vi "BezierGeneratorRev2Trans.vi"(1 "RobotY":dbl, 2 "RobotX":dbl, 3 "DeltaYaw":dbl, 4 "RobotOrientation":dbl=70.0, 5 "DeltaY":dbl=60.0, 6 "DeltaX":dbl=60.0) -> (0 "RobotNeededPathData":T1={"Path"=[], "MaxVel"=80.0, "MaxAccel"=100.0, "Backwards?"=FALSE, "PointSpacing"=6.0, "LookaheadDist"=13.0, "Speed/Curve"=1.8, "SlowDistanceAtEnd"=0.0, "SlowSpeed"=0.0, "MaxDeAccel"=80.0} {"SlowSpeed" format="%#_13g"; "SlowDistanceAtEnd" format="%#_13g"; "Speed/Curve" format="%#_13g"})   [LabVIEW 2018]
uses:
  FRC-2019-master/FRC-2019-master/Dawgma Programming Library/Controls/PurePursuit/RobotNeededPathData.ctl
panel:
  in  "SlowSpeed":dbl
  in  "SlowDistanceAtEnd":dbl
  in  "Speed/Curve":dbl=1.8
  in  "LookaheadDist":dbl=13.0
  in  "PointSpacing":dbl=6.0
  in  "MaxDeaccel":dbl=80.0
  in  "MaxAccel":dbl=100.0
  in  "MaxVel":dbl=80.0
  out "Curve":cluster{"X":dbl, "Y":dbl}[](graph)
  out "waypoints":cluster{dbl[], dbl[]}(graph)
  in  "TrajPointoffset":dbl=12.0
  in  "TargetOffset":dbl=12.0
  in  "Path":cluster{"x":dbl, "y":dbl}[](array[cluster])=[{"x"=0.0, "y"=0.0}, {"x"=0.0, "y"=0.0}, {"x"=0.0, "y"=0.0}, {"x"=0.0, "y"=0.0}]
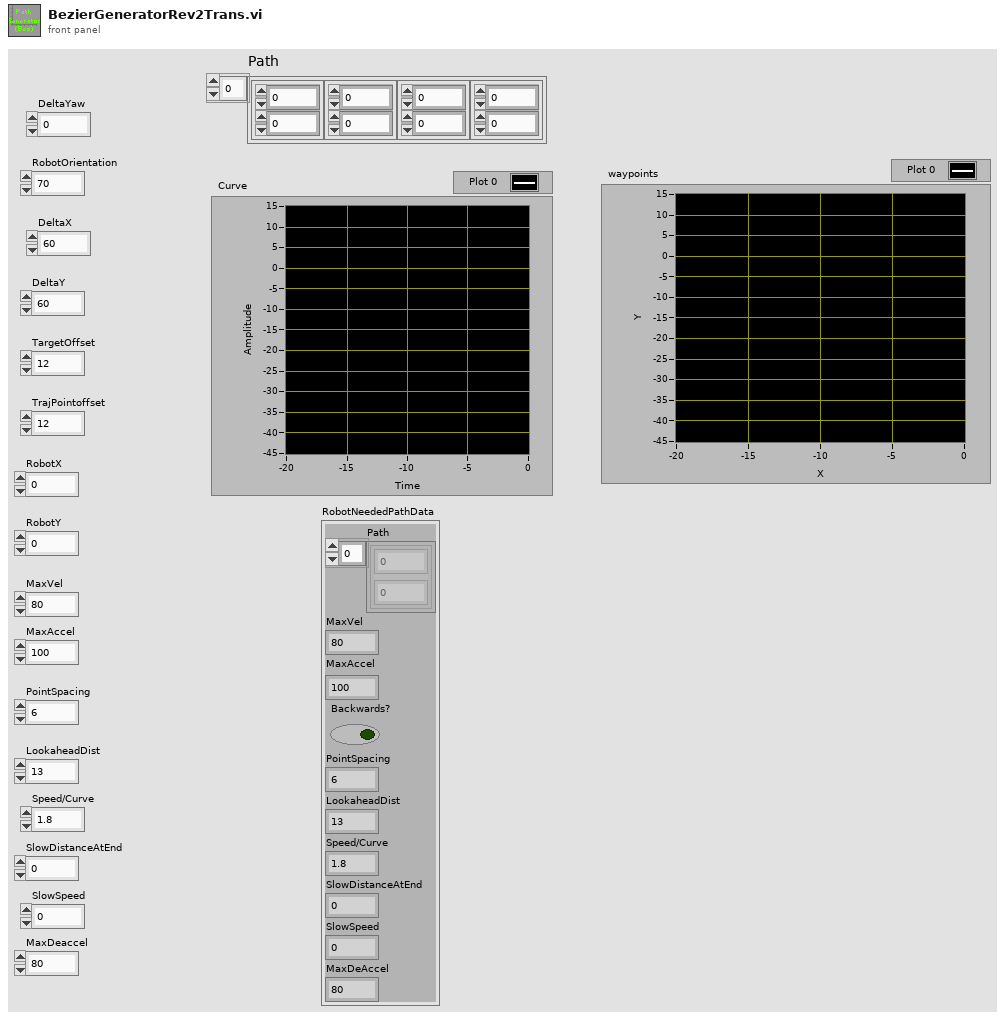
[diagram p1: front panel]
types:
  T1 = typedef "RobotNeededPathData.ctl" = cluster{"Path":cluster{dbl, dbl}[], "MaxVel":dbl, "MaxAccel":dbl, "Backwards?":bool, "PointSpacing":dbl, "LookaheadDist":dbl, "Speed/Curve":dbl, "SlowDistanceAtEnd":dbl, "SlowSpeed":dbl, "MaxDeAccel":dbl}
  T2 = cluster{"DeltaX":dbl, "DeltaY":dbl, "RobotOrientation":dbl, "TrajPointoffset":dbl, "TargetOffset":dbl, "DeltaYaw":dbl, "RobotX":dbl, "RobotY":dbl}
  T3 = cluster{cluster{"xP":dbl, "yP":dbl}[], "MaxVel":dbl, "MaxAccel":dbl, bool, "PointSpacing":dbl, "LookaheadDist":dbl, "Speed/Curve":dbl, "SlowDistanceAtEnd":dbl, "SlowSpeed":dbl, "MaxDeaccel":dbl}
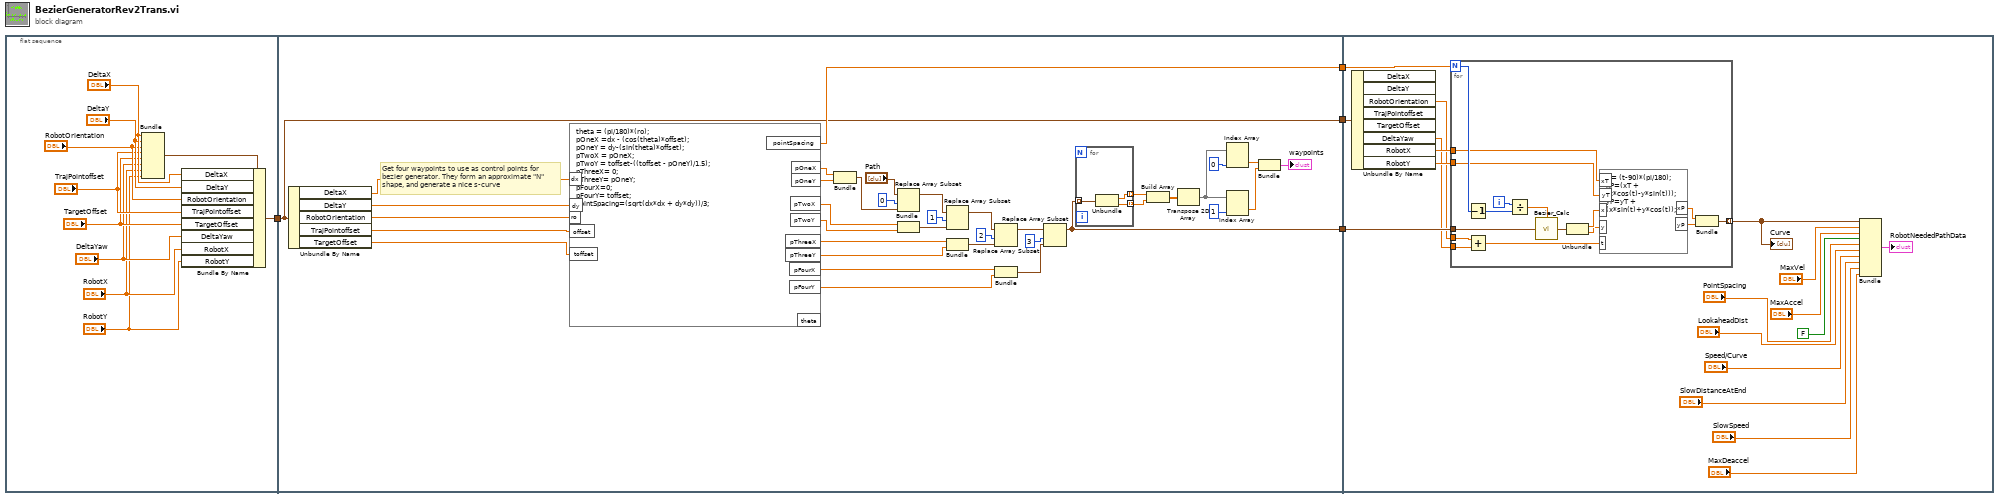
[diagram p0: block diagram]
diagram:
  n1 = flat-sequence {
    tunnel: [w13] -> w2
    tunnel: [w33] -> w4
    tunnel: [w22] -> w3
    tunnel: w2 -> [w15]
    tunnel: [w15] -> w1
    tunnel: w4 -> [w72]
    tunnel: w3 -> [w71]
    tunnel: w1 -> [w60]
    frame #0 {
      n2 = Bundle("DeltaX"="DeltaX", "DeltaY"="DeltaY", "RobotOrientation"="RobotOrientation", "TrajPointoffset"="TrajPointoffset", "TargetOffset"="TargetOffset", "DeltaYaw"="DeltaYaw", "RobotX"="RobotX", "RobotY"="RobotY") -> (w14:T2)  [unwired: 1 in]
      n3 = Bundle By Name(cluster=w14, "DeltaX"="DeltaX", "DeltaY"="DeltaY", "RobotOrientation"="RobotOrientation", "TrajPointoffset"="TrajPointoffset", "TargetOffset"="TargetOffset", "DeltaYaw"="DeltaYaw", "RobotX"="RobotX", "RobotY"="RobotY") -> (w13:T2)
    }
    frame #1 {
      # "Get four waypoints to use as control points for bezier generator. They form an approximate \"N\" shape, and generate a nice s-curve"
      n4 = Unbundle By Name(w15) -> ("DeltaX"=w27:dbl, "DeltaY"=w26:dbl, "RobotOrientation"=w23:dbl, "TrajPointoffset"=w24:dbl, "TargetOffset"=w25:dbl)
      n5 = formula code="theta = (pi/180)*(ro);\npOneX =dx - (cos(theta)*offset);\npOneY = dy-(sin(theta)*offset);\npTwoX = pOneX;\npTwoY = toffset-((toffset - pOneY)/1.5);\npThreeX= 0;\npThreeY= pOneY;\npFourX=0;\npFourY= toffset;\npointSpacing=(sqrt(dx*dx + dy*dy))/3;"("ro"=w23, "dx"=w27, "dy"=w26, "offset"=w24, "toffset"=w25) -> ("pOneX"=w31:dbl, "pOneY"=w30:dbl, "pTwoX"=w29:dbl, "pTwoY"=w28:dbl, "pointSpacing"=w22:dbl, "pThreeX"=w21:dbl, "pThreeY"=w20:dbl, "pFourX"=w19:dbl, "pFourY"=w18:dbl)  [unwired: 1 out]
      n6 = Bundle("pOneX"=w31, "pOneY"=w30) -> (w42:cluster{"pOneX":dbl, "pOneY":dbl})  [unwired: 1 in]
      n7 = Replace Array Subset(array="Path", new element=w42, index=0) -> (w48:cluster{"x":dbl, "y":dbl}[])
      n8 = Bundle("pTwoX"=w29, "pTwoY"=w28) -> (w43:cluster{"pTwoX":dbl, "pTwoY":dbl})  [unwired: 1 in]
      n9 = Replace Array Subset(array=w48, new element=w43, index=1) -> (w46:cluster{"x":dbl, "y":dbl}[])
      n10 = Bundle("pThreeX"=w21, "pThreeY"=w20) -> (w16:cluster{"pThreeX":dbl, "pThreeY":dbl})  [unwired: 1 in]
      n11 = Replace Array Subset(array=w46, new element=w16, index=2) -> (w44:cluster{"x":dbl, "y":dbl}[])
      n12 = Bundle("pFourX"=w19, "pFourY"=w18) -> (w17:cluster{"pFourX":dbl, "pFourY":dbl})  [unwired: 1 in]
      n13 = Replace Array Subset(array=w44, new element=w17, index=3) -> (w33:cluster{"x":dbl, "y":dbl}[])
      n14 = for {
        tunnel: w33 -> [w54] mode=indexing
        tunnel: [w53] -> w41 mode=indexing
        tunnel: [w52] -> w40 mode=indexing
        n15 = Unbundle(w54) -> ("x"=w53:dbl, "y"=w52:dbl)
      }
      n16 = Build Array(w41, w40) -> (w39:dbl[][])
      n17 = Transpose 2D Array(2D array=w39) -> (transposed array=w36:dbl[][])
      n18 = Index Array(array=w36, index (col)=0 ("disabled index (col)")) -> (element=w34:dbl[])  [unwired: 1 in]
      n19 = Index Array(array=w36, index (col)=1 ("disabled index (col)")) -> (element=w35:dbl[])  [unwired: 1 in]
      n20 = Bundle(w34, w35) -> (→"waypoints":cluster{dbl[], dbl[]})  [unwired: 1 in]
    }
    frame #2 {
      n21 = Unbundle By Name(w60) -> ("RobotOrientation"=w57:dbl, "DeltaYaw"=w56:dbl, "RobotX"=w59:dbl, "RobotY"=w58:dbl)  [unwired: 4 out]
      n22 = for {
        N: w71 -> [w88]
        tunnel: w72 -> [w84]
        tunnel: [w73] -> w55 mode=indexing
        tunnel: w59 -> [w83]
        tunnel: w58 -> [w82]
        tunnel: w57 -> [w78]
        tunnel: w56 -> [w77]
        i -> [w87]
        n23 = Decrement(x=w88) -> (x-1=w86:i32)
        n24 = Add(x=w78, y=w77) -> (x+y=w76:dbl)
        n25 = Divide(x=w87, y=w86) -> (x/y=w85:dbl)
        n26 = call "Bezier_Calc.vi"("points"=w84, "t"=w85) -> ("point out"=w81:cluster{"x":dbl, "y":dbl})
        n27 = Unbundle(w81) -> ("x"=w80:dbl, "y"=w79:dbl)
        n28 = formula code="t = (t-90)*(pi/180);\nxP=(xT + (x*cos(t)-y*sin(t)));\nyP=yT + (x*sin(t)+y*cos(t));"("x"=w80, "y"=w79, "t"=w76, "xT"=w83, "yT"=w82) -> ("yP"=w74:dbl, "xP"=w75:dbl)
        n29 = Bundle("xP"=w75, "yP"=w74) -> (w73:cluster{"xP":dbl, "yP":dbl})  [unwired: 1 in]
      }
      "Curve" <- w55
      n30 = Bundle(w55, "MaxVel"="MaxVel", "MaxAccel"="MaxAccel", FALSE, "PointSpacing"="PointSpacing", "LookaheadDist"="LookaheadDist", "Speed/Curve"="Speed/Curve", "SlowDistanceAtEnd"="SlowDistanceAtEnd", "SlowSpeed"="SlowSpeed", "MaxDeaccel"="MaxDeaccel") -> (→"RobotNeededPathData":T3)  [unwired: 1 in]
    }
  }
